vi "MAIN_csv_to_csv.vi"() -> ()   [LabVIEW 2017]
doc: "Permite obtener un archivo CSV de etiquetado automático de secciones de señal. \nIngresa: un archivo CSV que contiene el sample inicial, final y la etiqueta correspondiente.\nUn archivo TDMS que contenga la información del registro de la señal.\nSe debe colocar la dirección del archivo de salida.\nEstablecer el número de samples que contendrá cada parte en que se dividirá la sección.\nAl momento el VI no contempla traslapamiento."
uses:
  <vilib>/Waveform/WDTOps.llb/WDT Get Waveform Subset DBL.vi
  <vilib>/addons/Sound and Vibration/svt_Octave_2014 standard/SVT Third-octave Analysis (1 Ch).vi
  <vilib>/Utility/file.llb/Write Delimited Spreadsheet (string).vi
  <vilib>/addons/Sound and Vibration/svt_Octave/SoundVib_Octave_2014 standard.lvlib
panel:
  in  "Canal":string[](array[string])=["Sound Pressure_0"]
  out "Para el CSV, excepto fecha y hora":string[][](array[string])
  out "TIEMPOS":timestamp[](array[timestamp])
  out "Objetos por sección.":i32[][](array[numeric])
  out "Objetos":i32[](array[numeric])
  out "Secciones":i32[](array[numeric])
  out "Objetos totales":i32
  in  "frequency range":T1={"low band"=enum."20 Hz", "high band"=enum."20000 Hz"}
  out "TO CSV.":string[][](array[string])
  out "ETIQUETAS":string[](array[string])
  out "BANDAS":dbl[][](array[numeric])
  in  "ETIQUETADO":path=path "C:/Users/CRamos/Documents/MATLAB/etiquetador/csv_OUT/DATOS_caracte.csv"
  out "Objeto actual":i32
  out "Sección Actual":i32
  out "Samples \npor Objeto":waveform(dbl)
  in  "Largo de ventada temporal en N samples":dbl=4410.0
  out "Secciones":waveform(dbl)[](array[waveform])
  out "Multiplot \noctave graph":T2(graph)
  in  "ARCHIVO\nTDMS":path=path "C:/Users/CRamos/Documents/MATLAB/TDMS_files/two_sounds.tdms"
  in  "Archivo de\nreferencias (.csv)":path=path "C:/Users/CRamos/Documents/MATLAB/etiquetador/csv_IN/DATOS.csv"
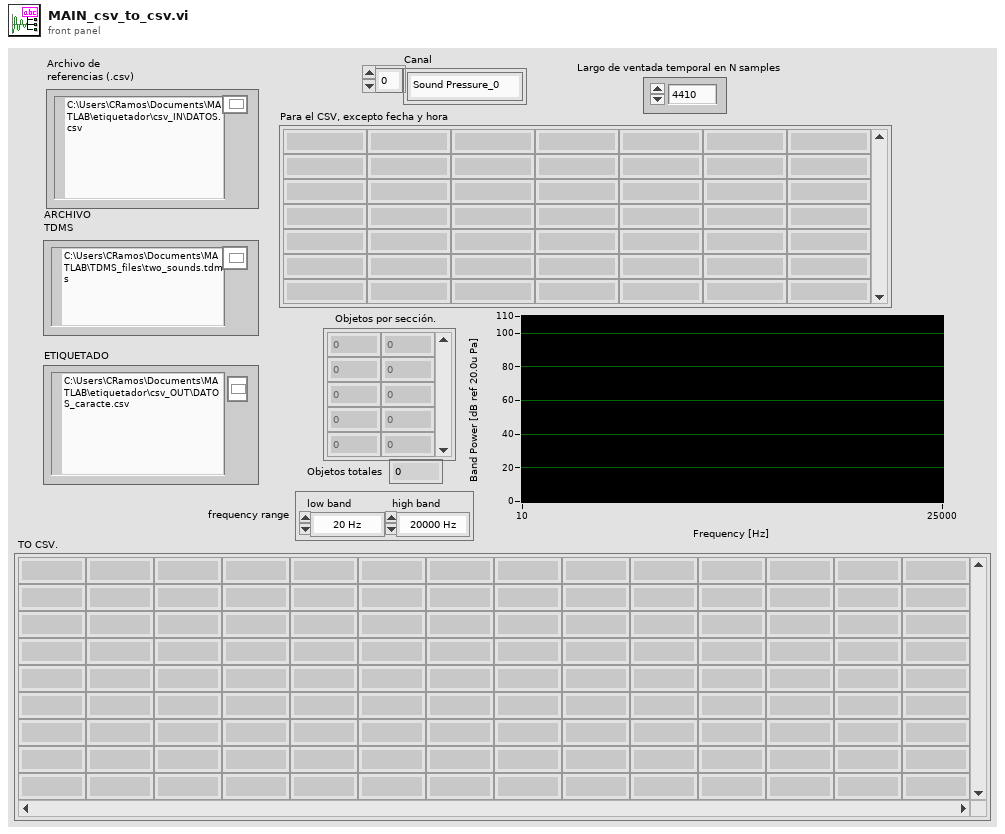
[diagram p1: front panel]
types:
  T1 = cluster{"low band":enum16{"20 Hz", "25 Hz", "31.5 Hz", "40 Hz", "50 Hz", "63 Hz", "80 Hz", "100 Hz", "125 Hz", "160 Hz", "200 Hz", "250 Hz", "315 Hz", "400 Hz", "500 Hz", "630 Hz", "800 Hz", "1000 Hz", "1250 Hz", "1600 Hz", "2000 Hz", "2500 Hz", "3150 Hz", "4000 Hz", "5000 Hz", "6300 Hz", "8000 Hz", "10000 Hz", "12500 Hz", "16000 Hz", "20000 Hz"}, "high band":enum16{"20 Hz", "25 Hz", "31.5 Hz", "40 Hz", "50 Hz", "63 Hz", "80 Hz", "100 Hz", "125 Hz", "160 Hz", "200 Hz", "250 Hz", "315 Hz", "400 Hz", "500 Hz", "630 Hz", "800 Hz", "1000 Hz", "1250 Hz", "1600 Hz", "2000 Hz", "2500 Hz", "3150 Hz", "4000 Hz", "5000 Hz", "6300 Hz", "8000 Hz", "10000 Hz", "12500 Hz", "16000 Hz", "20000 Hz"}}
  T2 = cluster{"nominal frequencies [Hz]":dbl[], "band power":dbl[]}
  T3 = enum16{"open", "open or create", "create or replace", "create", "open (read-only)"}
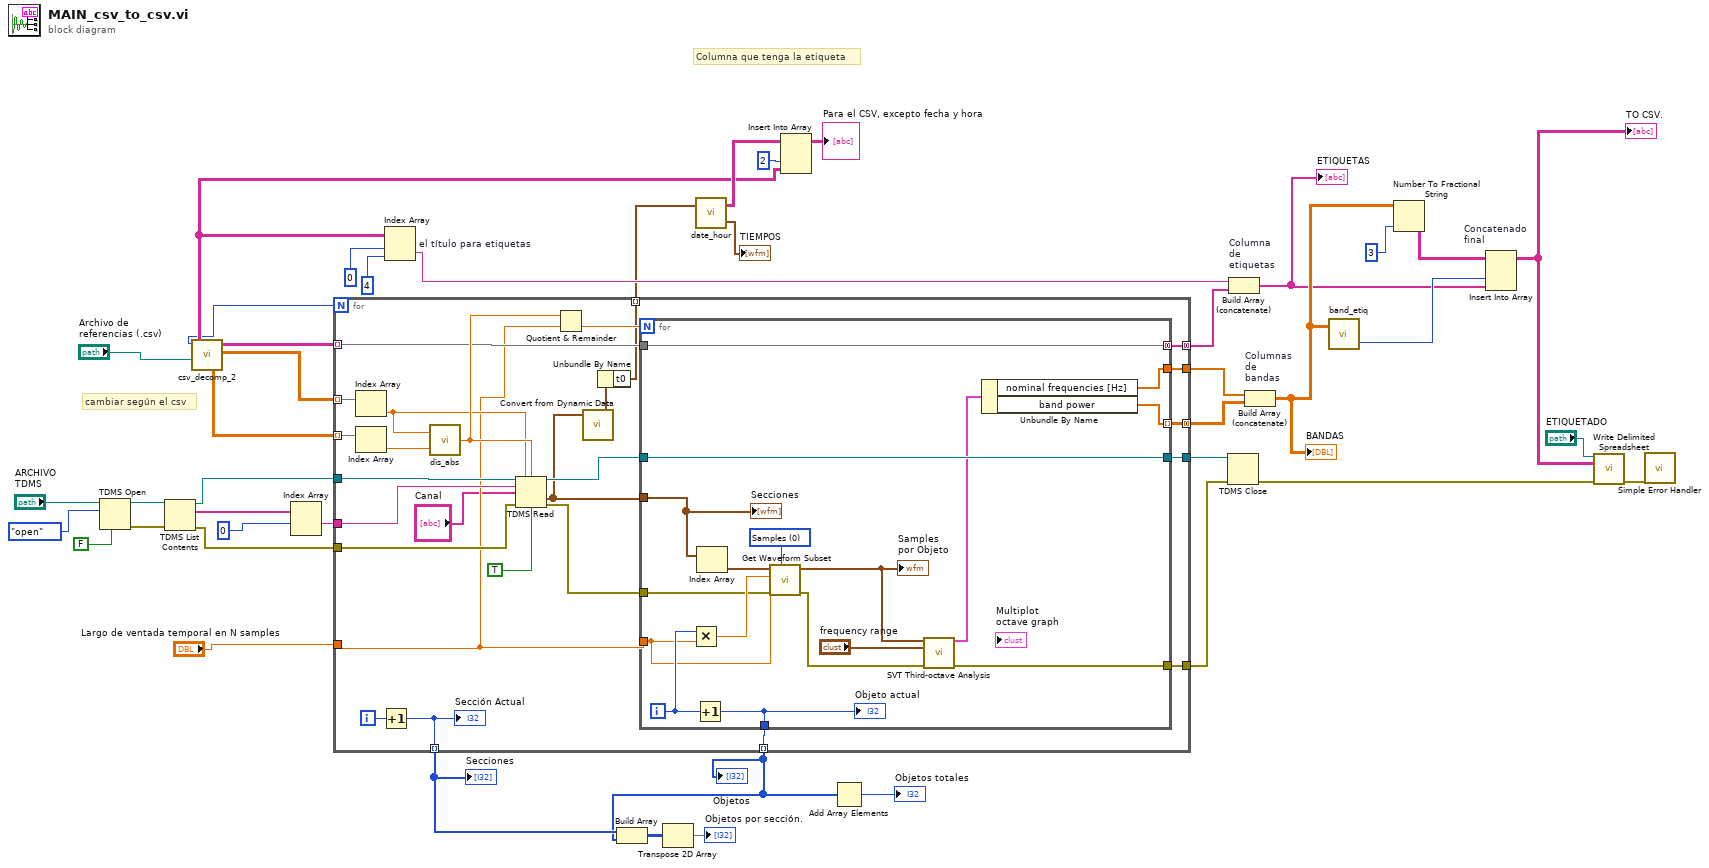
[diagram p0: block diagram]
diagram:
  # "cambiar según el csv"
  # "Columna que tenga la etiqueta"
  n1 = TDMS Open(6:FALSE ("disable buffering? (T)"), 10:T3."open" ("operation (0:open)"), 11:"ARCHIVO\nTDMS") -> (0:w41:errorcluster, 3:w9:refnum<k34>)  [unwired: 4 in]
  n2 = TDMS List Contents(4:w41, 7:w9) -> (0:w7:errorcluster, 2:w8:string[], 3:w40:refnum<k34>)  [unwired: 1 in, 1 out]
  n3 = call "csv_decomp_2.vi"("Archivo de referencias (.csv)"="Archivo de\nreferencias (.csv)") -> ("finales"=w2:dbl[][], "iniciales"=w1:dbl[][], "etiquetas"=w3:string[][], "# dimención"=w4:i32, "Lectura CSV"=w6:string[][])  [unwired: 2 in]
  n4 = Index Array(array=w8, index #1=0 ("index")) -> (element #1=w38:string)  [unwired: 1 in, 1 out]
  n5 = for {
    N: w4 -> [_]
    tunnel: w1 -> [w67] mode=indexing
    tunnel: w2 -> [w68] mode=indexing
    tunnel: w3 -> [w55] mode=indexing
    tunnel: w40 -> [w69]
    tunnel: w7 -> [w62]
    tunnel: w38 -> [w70]
    tunnel: [w60] -> w37
    tunnel: [w58] -> w36
    tunnel: [w57] -> w35 mode=concatenating
    tunnel: [w56] -> w33
    tunnel: [w54] -> w30 mode=concatenating
    tunnel: [w53] -> w17 mode=indexing
    tunnel: "Largo de ventada temporal en N samples" -> [w50]
    tunnel: [w49] -> w18 mode=indexing
    tunnel: [w46] -> w14 mode=indexing
    i -> [w59]
    n6 = Index Array(array=w67) -> (element=w52:dbl)  [unwired: 1 in]
    n7 = Index Array(array=w68) -> (element=w51:dbl)  [unwired: 1 in]
    n8 = Increment(x=w59) -> (x+1=w49:i32)
    "Sección Actual" <- w49
    n9 = call "dis_abs.vi"("Numeric in"=w51, "Numeric 3"=w52) -> ("distancia abs entre dos números"=w63:dbl)
    n10 = TDMS Read(0:w69, 1:w52, 2:w63, 5:w70, 7:"Canal", 11:w62, 13:TRUE ("return channels in file order? (F)")) -> (4:w66:refnum<k34>, 10:w48:waveform(dbl)[], 15:w61:errorcluster)  [unwired: 1 in, 3 out]
    n11 = Quotient & Remainder(x=w63, y=w50) -> (floor(x/y)=w64:dbl)  [unwired: 1 out]
    n12 = call "Convert from Dynamic Data"("Dynamic Data Type"=w48) -> ("Waveform"=w47:waveform(dbl))  [unwired: 3 in]
    n13 = Unbundle By Name(w47) -> ("t0"=w46:timestamp)
    n14 = for {
      N: w64 -> [_]
      tunnel: w66 -> [w80]
      tunnel: w48 -> [w72]
      tunnel: w61 -> [w82]
      tunnel: [w81] -> w56
      tunnel: [w80] -> w60
      tunnel: [w79] -> w58
      tunnel: [w78] -> w57 mode=indexing
      tunnel: w55 -> [w77]
      tunnel: [w77] -> w54 mode=concatenating
      tunnel: [w75] -> w53
      tunnel: w50 -> [w73]
      i -> [w74]
      w85 = u16 0 items=["Samples", "Relative Time"] ("start/duration format")
      n15 = Multiply(x=w74, y=w73) -> (x*y=w83:dbl)
      n16 = Increment(x=w74) -> (x+1=w75:i32)
      "Objeto actual" <- w75
      n17 = Index Array(array=w72) -> (element=w86:waveform(dbl))  [unwired: 1 in]
      n18 = call-poly <vilib>:"Get Waveform Subset.vi"("start/duration format"=w85, "error in (no error)"=w82, "duration"=w73, "start samples/time"=w83, "waveform in"=w86) -> ("error out"=w87:errorcluster, "waveform out"=w84:waveform(dbl))  [unwired: 1 in, 2 out]
      "Samples \npor Objeto" <- w84
      n19 = call-poly <vilib>:"SVT Third-octave Analysis.vi"("scaled signal [EU]"=w84, "frequency range"="frequency range", "error in (no error)"=w87) -> ("octave spectrum"=w71:T2, "error out"=w81:errorcluster)  [unwired: 7 in, 4 out]
      n20 = Unbundle By Name(w71) -> ("nominal frequencies [Hz]"=w79:dbl[], "band power"=w78:dbl[])
      "Secciones" <- w72
    }
  }
  "Secciones" <- w18
  "Objetos" <- w17
  n21 = Index Array "el título para etiquetas"(array=w6, index (row)=0 ("disabled index (row)"), index (col)=4 ("disabled index (col)")) -> (element=w27:string)
  n22 = Build Array(w18, w17) -> (w16:i32[][])
  n23 = Transpose 2D Array(2D array=w16) -> (transposed array=→"Objetos por sección.":i32[][])
  n24 = call "date_hour.vi"("Array"=w14) -> ("date/hour"=→"TIEMPOS":timestamp[], "appended array"=w12:string[][])  [unwired: 1 in]
  n25 = Insert Into Array(array=w12, index (col)=2 ("disabled index (col)"), new element=w6) -> (→"Para el CSV, excepto fecha y hora":string[][])  [unwired: 1 in]
  n26 = Add Array Elements(numeric array=w17) -> (sum=→"Objetos totales":i32)
  n27 = TDMS Close(8:w33, 11:w37) -> (0:w32:errorcluster)  [unwired: 1 out]
  n28 = Build Array (concatenate) "Columna \nde \netiquetas"(w27, w30) -> (w21:string[])
  "ETIQUETAS" <- w21
  n29 = Build Array (concatenate) "Columnas \nde\nbandas"(w36, w35) -> (w24:dbl[][])
  "BANDAS" <- w24
  n30 = call "band_etiq.vi"("Array de entrada"=w24) -> ("Numeric"=w23:i32)  [unwired: 1 in, 1 out]
  n31 = Number To Fractional String(number=w24, precision (6)=i16 3) -> (F-format string=w25:string[][])  [unwired: 2 in]
  n32 = Insert Into Array "Concatenado \nfinal"(array=w25, index (col)=w23, new element=w21) -> (w22:string[][])  [unwired: 1 in]
  "TO CSV." <- w22
  n33 = call-poly <vilib>:"Write Delimited Spreadsheet.vi"("file path (dialog if empty)"="ETIQUETADO", "2D data"=w22, "error in (no error)"=w32) -> ("error out"=w31:errorcluster)  [unwired: 11 in, 1 out]
  n34 = call <vilib>:"Simple Error Handler.vi"("error in (no error)"=w31) -> ()  [unwired: 4 in, 5 out]
